vi "SaveForPrevious.vi"() -> ()   [LabVIEW 2019]
panel:
  out "error out":errorcluster
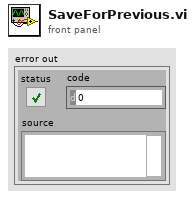
[diagram p1: front panel]
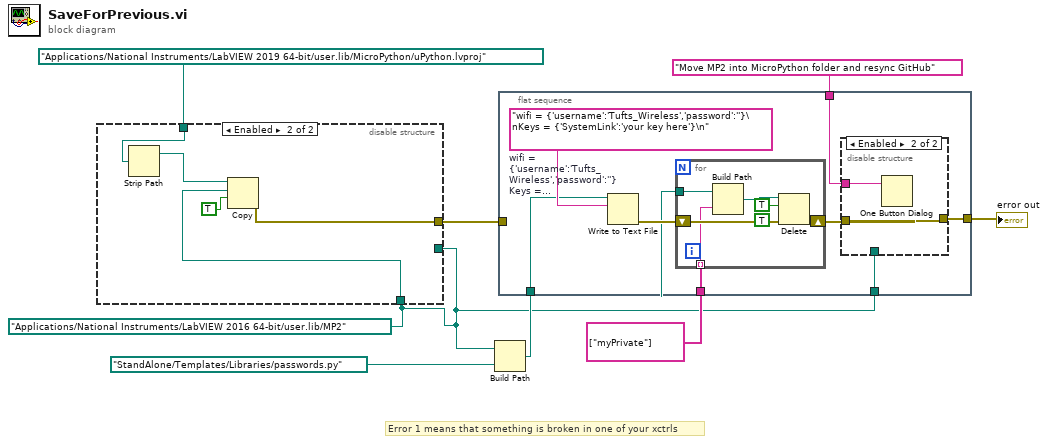
[diagram p0: block diagram]
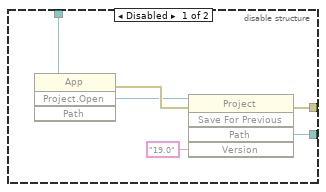
[diagram p2: hidden frame]
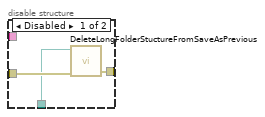
[diagram p3: hidden frame]
diagram:
  w1 = path "/Applications/National Instruments/LabVIEW 2016 64-bit/user.lib/MP2" ("Path")
  # "Error 1 means that something is broken in one of your xctrls"
  n1 = disable-structure shown="Enabled" {
    disable-tunnel: [w11 w15] -> w7
    disable-tunnel: path "/Applications/National Instruments/LabVIEW 2019 64-bit/user.lib/MicroPython/uPython.lvproj" ("Path") -> [w10 w19]
    disable-tunnel: w1 -> [w9 _]
    disable-tunnel: w1 -> [_ w16]
    frame Disabled {
      n2 = invoke class="App" method="Project.Open"("Path"=w10) -> (error out=w14:errorcluster, "Project:Open"=w13:refnum<vi>)  [unwired: 3 in, 2 out]
      n3 = invoke class="Project" method="Save For Previous"(reference=w13, error in=w14, "Path"=w9, "Version"="19.0") -> (error out=w11:errorcluster)  [unwired: 1 in, 4 out]
    }
    frame Enabled {
      n4 = Strip Path(path=w19) -> (stripped path=w17:path)  [unwired: 1 out]
      n5 = Copy(9:TRUE ("overwrite (F)"), 10:w16, 11:w17) -> (0:w15:errorcluster)  [unwired: 2 in, 2 out]
    }
  }
  n6 = Build Path(base path=w1, name or relative path=path "StandAlone/Templates/Libraries/passwords.py" ("Path")) -> (appended path=w5:path)
  n7 = flat-sequence {
    tunnel: [w27] -> w8
    tunnel: w7 -> [_]
    tunnel: w5 -> [w25]
    tunnel: w1 -> [w23]
    tunnel: string[] ["myPrivate"] -> [w21]
    tunnel: "Move MP2 into MicroPython folder and resync GitHub" -> [w20]
    frame #0 {
      w26 = "wifi = {'username':'Tufts_Wireless','password':''}\nKeys = {'SystemLink':'your key here'}\n"  # wifi = {'username':'Tufts_Wireless','password':''} Keys = {'SystemLink':'your key here'}
      n8 = Write to Text File(file (use dialog)=w25, text=w26) -> (error out=w24:errorcluster)  [unwired: 2 in, 2 out]
      n9 = for {
        tunnel: w23 -> [w33]
        tunnel: w21 -> [w28] mode=indexing
        shift-right: [w29] -> w22
        shift-left: w24 -> [w34]
        n10 = Build Path(base path=w33, name or relative path=w28) -> (appended path=w32:path)
        n11 = Delete(path (use dialog)=w32, entire hierarchy (F)=TRUE, confirm (F)=TRUE, error in=w34) -> (error out=w29:errorcluster)  [unwired: 1 in, 2 out]
      }
      n12 = disable-structure shown="Enabled" {
        disable-tunnel: [w37 w39] -> w27
        disable-tunnel: w22 -> [w36 w39]
        disable-tunnel: w23 -> [w35 _]
        disable-tunnel: w20 -> [_ w38]
        frame Disabled {
          n13 = call <userlib>:"DeleteLongFolderStuctureFromSaveAsPrevious.vi"("error in"=w36, "Path"=w35) -> ("error out"=w37:errorcluster)  [unwired: 9 in]
        }
        frame Enabled {
          n14 = One Button Dialog(message=w38) -> ()  [unwired: 1 in, 1 out]
        }
      }
    }
  }
  "error out" <- w8
